vi "axis.vi"(0 "origin":cluster{"X":sgl, "Y":sgl, "Z":sgl}={"X"=1.0, "Y"=0.0, "Z"=0.0}) -> (4 "urdf out":string)   [LabVIEW 2010]
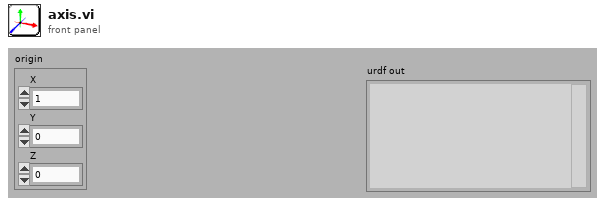
[diagram p1: front panel]
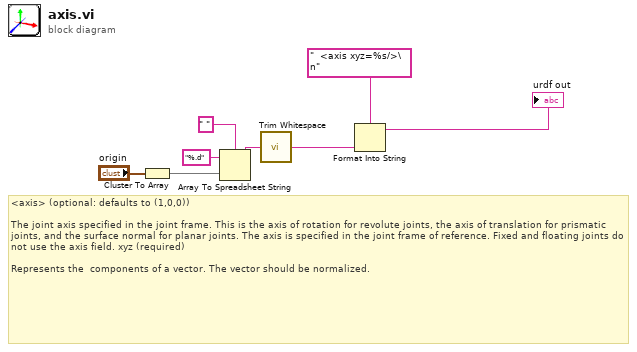
[diagram p0: block diagram]
diagram:
  # "<axis> (optional: defaults to (1,0,0))\n\nThe joint axis specified in the joint frame. This is the axis of rotation for revolute joints, the axis of translation for prismatic joints, and the surface normal for planar joints. The axis is specified in the joint frame of reference. Fixed and floating joints do not use the axis field. xyz (required) \n\nRepresents the  components of a vector. The vector should be normalized."
  n1 = Cluster To Array(cluster="origin") -> (array=w7:sgl[])
  n2 = Array To Spreadsheet String(delimiter (Tab)=" ", array=w7, 3:"%.d" ("format string")) -> (spreadsheet string=w4:string)
  n3 = call <vilib>:"Trim Whitespace.vi"("string"=w4) -> ("trimmed string"=w1:string)  [unwired: 1 in]
  n4 = Format Into String(format string="  <axis xyz=%s/>\n", w1) -> (resulting string=→"urdf out":string)  [unwired: 2 in, 1 out]
